vi "Sweep Reset.vi"(8 "error in (no error)":errorcluster, 9 "Sweep outfile":path, 10 "addr":i32, 11 "instrument handle":refnum<k15>) -> (0 "error out":errorcluster, 1 "final current (A)":dbl, 2 "final resistance (ohm)":dbl, 3 "instrument handle out":refnum<k15>)   [LabVIEW 2018]
uses:
  <instrlib>/niDigital/niDigital.llb/niDigital Burst Pattern (Burst Only).vi
  <vilib>/Utility/file.llb/Write Delimited Spreadsheet (DBL).vi
panel:
  out "WL voltage (V)":dbl
  out "SL voltage (V)":dbl
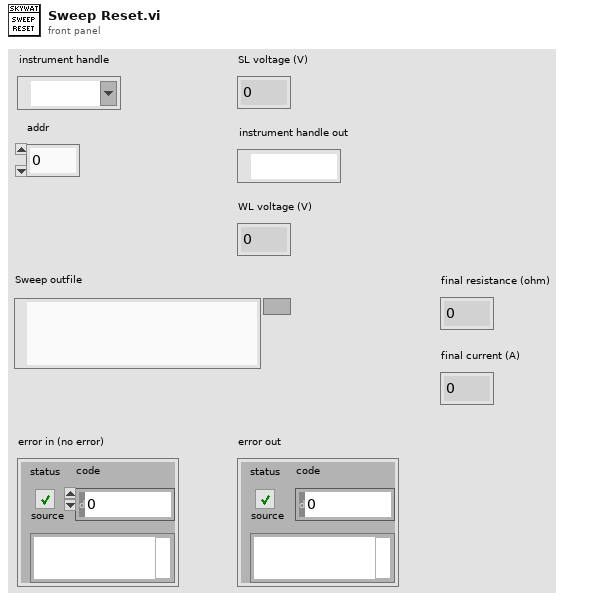
[diagram p1: front panel]
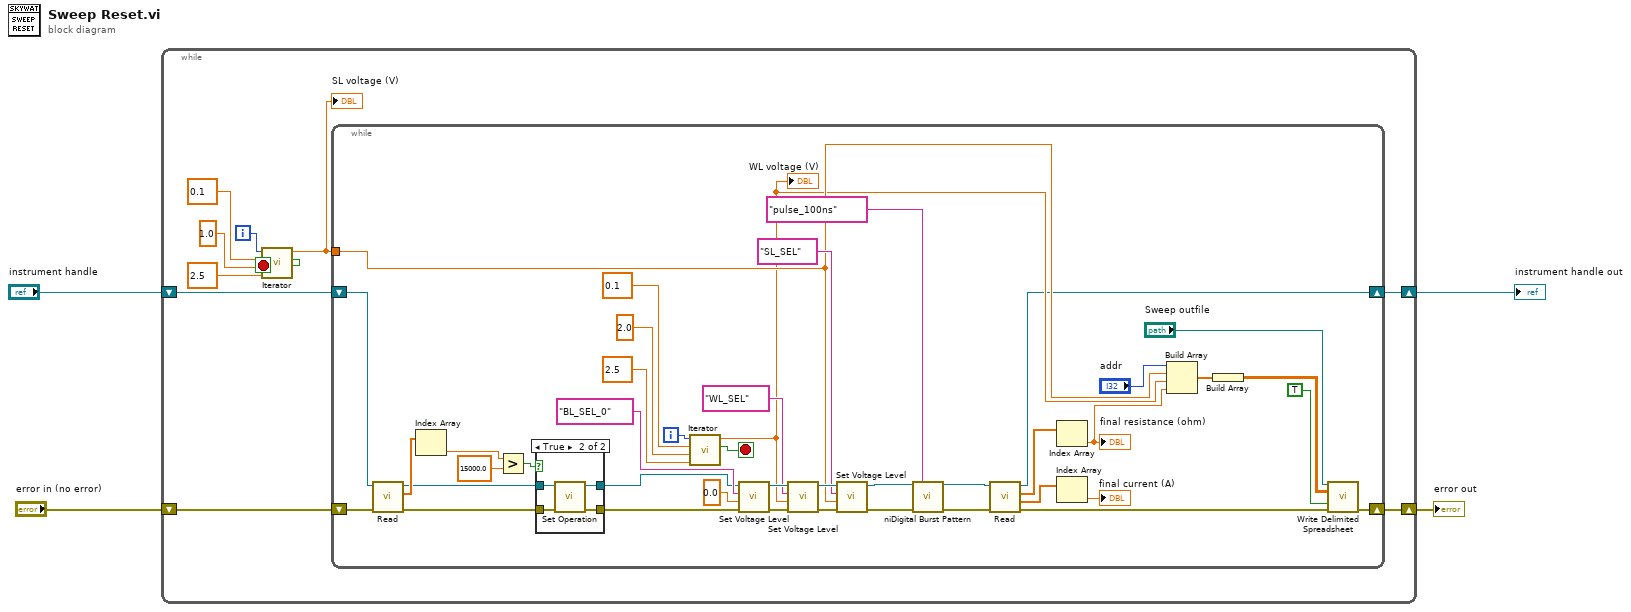
[diagram p0: block diagram]
diagram:
  n1 = while {
    shift-right: [w11] -> w4
    shift-left: "instrument handle" -> [w9]
    shift-right: [w10] -> w1
    shift-left: "error in (no error)" -> [w8]
    i -> [w12]
    stop <- w5 stop-if-true
    n2 = call "Iterator.vi"("Final Value"=2.5 ("y"), "Initial Value"=1.0 ("y"), "Step"=0.1 ("x"), "i"=w12) -> ("End Loop"=w5:bool, "Current Value"=w6:dbl)  [unwired: 6 in]
    "SL voltage (V)" <- w6
    n3 = while {
      shift-right: [w20] -> w11
      shift-left: w9 -> [w51]
      shift-right: [w27] -> w10
      shift-left: w8 -> [w50]
      tunnel: w6 -> [w26]
      i -> [w56]
      stop <- w52 stop-if-true
      n4 = call "Read.vi"("error in (no error)"=w50, "instrument handle"=w51) -> ("error out"=w45:errorcluster, "resistances (ohm)"=w49:dbl[], "instrument handle out"=w46:refnum<k15>)  [unwired: 6 in, 1 out]
      n5 = Index Array(array=w49) -> (element=w18:dbl)  [unwired: 1 in]
      n6 = Greater?(x=w18, y=15000.0) -> (0:w47:bool)
      n7 = case shown="True" w47 {
        tunnel: w46 -> [w58 w62]
        tunnel: w45 -> [w57 w61]
        tunnel: [w58 w60] -> w36
        tunnel: [w57 w59] -> w35
        frame False {
        }
        frame True {
          n8 = call "Set Operation.vi"("error in (no error)"=w61, "instrument handle"=w62) -> ("error out"=w59:errorcluster, "instrument handle out"=w60:refnum<k15>)  [unwired: 8 in]
        }
      }
      n9 = call "Iterator.vi"("Final Value"=2.5 ("y"), "Initial Value"=2.0 ("y"), "Step"=0.1 ("x"), "i"=w56) -> ("End Loop"=w52:bool, "Current Value"=w25:dbl)  [unwired: 6 in]
      "WL voltage (V)" <- w25
      n10 = call "Set Voltage Level.vi"("error in (no error)"=w35, "level (V)"=0.0, "channel list"="BL_SEL_0", "instrument handle"=w36) -> ("error out"=w41:errorcluster, "instrument handle out"=w42:refnum<k15>)  [unwired: 6 in]
      n11 = call "Set Voltage Level.vi"("error in (no error)"=w41, "level (V)"=w25, "channel list"="WL_SEL", "instrument handle"=w42) -> ("error out"=w44:errorcluster, "instrument handle out"=w43:refnum<k15>)  [unwired: 6 in]
      n12 = call "Set Voltage Level.vi"("error in (no error)"=w44, "level (V)"=w26, "channel list"="SL_SEL", "instrument handle"=w43) -> ("error out"=w33:errorcluster, "instrument handle out"=w32:refnum<k15>)  [unwired: 6 in]
      n13 = call-poly <instrlib>:"niDigital Burst Pattern.vi"("instrument handle"=w32, "start label"="pulse_100ns", "error in"=w33) -> ("instrument handle out"=w21:refnum<k15>, "error out"=w23:errorcluster)  [unwired: 11 in]
      n14 = call "Read.vi"("error in (no error)"=w23, "instrument handle"=w21) -> ("error out"=w22:errorcluster, "currents (A)"=w16:dbl[], "resistances (ohm)"=w19:dbl[], "instrument handle out"=w20:refnum<k15>)  [unwired: 6 in]
      n15 = Index Array(array=w19) -> (element=w17:dbl)  [unwired: 1 in]
      "final resistance (ohm)" <- w17
      n16 = Index Array(array=w16) -> (element=→"final current (A)":dbl)  [unwired: 1 in]
      n17 = Build Array("addr", w26, w25, w17) -> (w29:dbl[])
      n18 = Build Array(w29) -> (w31:dbl[][])
      n19 = call-poly <vilib>:"Write Delimited Spreadsheet.vi"("file path (dialog if empty)"="Sweep outfile", "2D data"=w31, "append to file? (new file:F)"=TRUE, "error in (no error)"=w22) -> ("error out"=w27:errorcluster)  [unwired: 10 in, 1 out]
    }
  }
  "error out" <- w1
  "instrument handle out" <- w4
